vi "TDLAS1.vi"() -> ()   [LabVIEW 2016]
uses:
  <vilib>/DAQmx/read.llb/DAQmx Read (Analog DBL 1Chan 1Samp).vi
  <vilib>/DAQmx/create/channels.llb/DAQmx Create Channel (AI-Voltage-Basic).vi
  <vilib>/DAQmx/configure/timing.llb/DAQmx Timing (Sample Clock).vi
  <vilib>/DAQmx/miscellaneous.llb/DAQmx Fill In Error Info.vi
panel:
  in  "rate":dbl=1000.0 format="%0.2f"
  out "error out":errorcluster
  in  "stop":bool
  out "Waveform Chart":dbl(graph)
  out "data":dbl format="%0.2f"
  in  "timeout":dbl=10.0 format="%0.2f"
  in  "samples per channel":i32=1000
  in  "sample mode":i32(ring)=10178 items=["Finite Samples"=10178, "Continuous Samples"=10123, "Hardware Timed Single Point"=12522]
  in  "input terminal configuration":i32(ring)=-1 items=["Default"=-1, "RSE"=10083, "NRSE"=10078, "Differential"=10106, "Pseudodifferential"=12529]
  in  "minimum value":dbl=-5.0 format="%0.2f"
  in  "maximum value":dbl=5.0 format="%0.2f"
  in  "physical channels":tag
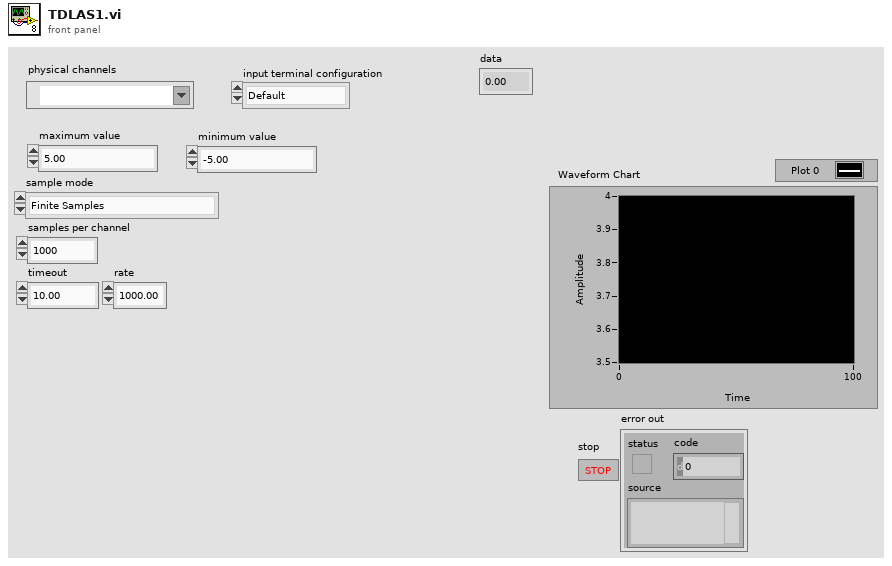
[diagram p1: front panel]
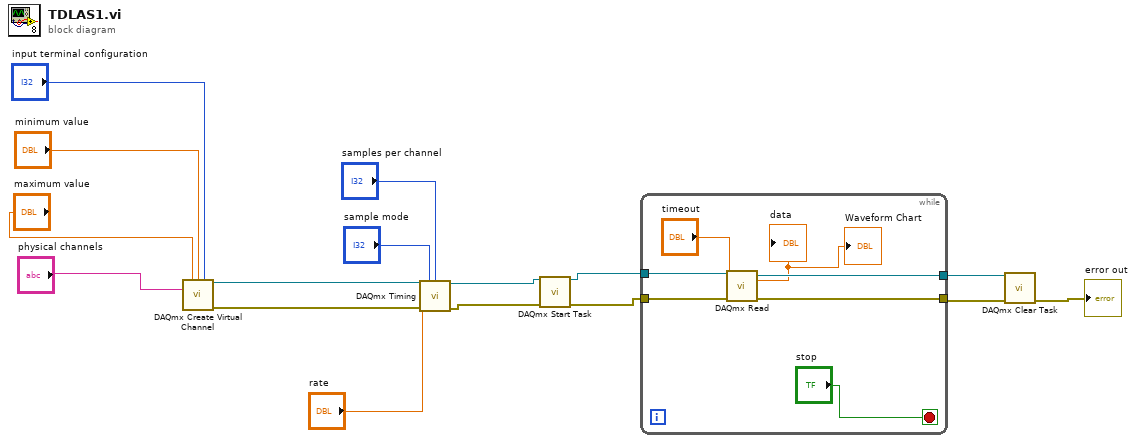
[diagram p0: block diagram]
diagram:
  n1 = call-poly <vilib>:"DAQmx Create Virtual Channel.vi"("maximum value"="maximum value", "minimum value"="minimum value", "input terminal configuration"="input terminal configuration", "physical channels"="physical channels") -> ("task out"=w12:refnum<k21>, "error out"=w11:errorcluster)  [unwired: 10 in]
  n2 = call-poly <vilib>:"DAQmx Timing.vi"("task/channels in"=w12, "sample mode"="sample mode", "samples per channel"="samples per channel", "rate"="rate", "error in"=w11) -> ("task out"=w8:refnum<k21>, "error out"=w7:errorcluster)  [unwired: 9 in]
  n3 = call <vilib>:"DAQmx Start Task.vi"("task/channels in"=w8, "error in"=w7) -> ("task out"=w6:refnum<k21>, "error out"=w5:errorcluster)  [unwired: 12 in]
  n4 = while {
    tunnel: w6 -> [w23]
    tunnel: w5 -> [w22]
    tunnel: [w20] -> w3
    tunnel: [w18] -> w4
    stop <- "stop" stop-if-true
    n5 = call-poly <vilib>:"DAQmx Read.vi"("task/channels in"=w23, "timeout"="timeout", "error in"=w22) -> ("task out"=w18:refnum<k21>, "data"=→"data" →"Waveform Chart":dbl, "error out"=w20:errorcluster)  [unwired: 10 in]
  }
  n6 = call <vilib>:"DAQmx Clear Task.vi"("task in"=w4, "error in"=w3) -> ("error out"=→"error out":errorcluster)  [unwired: 13 in]
